vi "Close_Shot.vi"(4 "Far Shot":bool, 6 "Low_Goal":bool, 7 "Servo_Ref":T4={"ServoDeviceRef"={"DeviceStatus"={"status"=FALSE, "code"=0, "source"=""}, "PWM Channel"=enum."PWM 9", "DeadBand"={"Name"="Servo", "maxPositivePwm"=1770, "minPositivePwm"=1013, "centerPwm"=1007, "maxNegativePwm"=1000, "minNegativePwm"=243, "angularRange"=170}}, "error out"={"status"=FALSE, "code"=0, "source"=""}}, 8 "Close_Shot":bool) -> (0 "Shooter_Motor":dbl=1.0, 1 "Shooter_Arm":T5=enum."Out", 2 "Stage_Motor":T6=enum."Off", 3 "Shooter_Active":bool)   [LabVIEW 2015]
uses:
  Motor_Dir_Type_Def.ctl
  Arm_defense_Type_Def.ctl
  <vilib>/Rock Robotics/WPI/PWM/Servo/WPI_ServoDeviceRef.ctl
  <vilib>/Rock Robotics/SystemInterfaces/DIO/FPGA_DIOPWMChannel.ctl
  <vilib>/Rock Robotics/WPI/PWM/WPI_PWMDeadband.ctl
  Global_Var/Drive_Global.vi
  <vilib>/addons/control/pid/pid.llb/PID (DBL).vi
  <vilib>/Rock Robotics/Network Tables/NT Read Boolean.vi
  <vilib>/Rock Robotics/Network Tables/NT Read Number.vi
  <vilib>/Rock Robotics/Network Tables/NT Write Number.vi
  <vilib>/addons/control/pid/NI_PID_pid.lvlib
panel:
  in  "Low_Goal_WHeel_Speed":dbl=0.4
  in  "Far Angle":dbl=180.0
  in  "Dashboard_Enable":bool
  in  "Negate":bool=TRUE
  out "Waveform Chart":cluster{"Shooter_Speed":dbl, "output":dbl}(graph)={"Shooter_Speed"=0.85, "output"=0.6528102795997961}
  in  "PID gains":T7={"proportional gain (Kc)"=5.0, "integral time (Ti, min)"=0.01, "derivative time (Td, min)"=0.0} {"derivative time (Td, min)" format="%.3f"; "integral time (Ti, min)" format="%.3f"; "proportional gain (Kc)" format="%.3f"}
  in  "Shooter_Speed":dbl=0.85
  in  "Shooter_PID_Enable":bool=TRUE
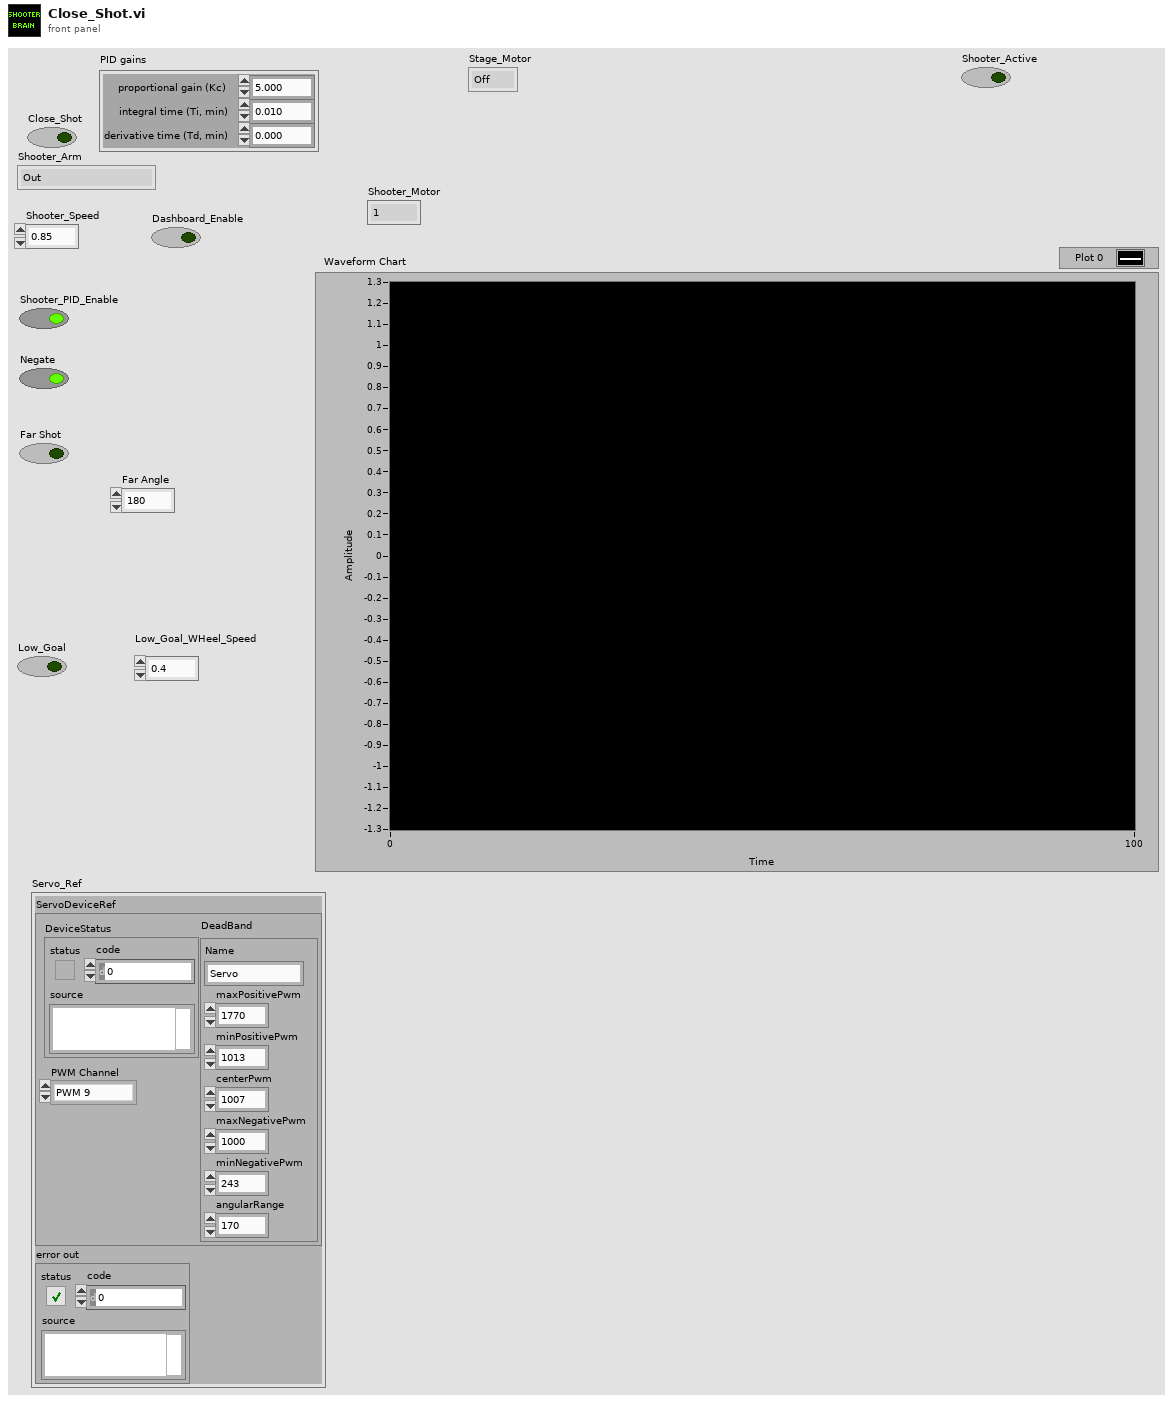
[diagram p1: front panel]
types:
  T1 = typedef "WPI_ServoDeviceRef.ctl" = cluster{"DeviceStatus":errorcluster, "PWM Channel":T2, "DeadBand":T3}
  T2 = typedef "FPGA_DIOPWMChannel.ctl" = enum8{"PWM 0", "PWM 1", "PWM 2", "PWM 3", "PWM 4", "PWM 5", "PWM 6", "PWM 7", "PWM 8", "PWM 9", "PWM MXP 0", "PWM MXP 1", "PWM MXP 2", "PWM MXP 3", "PWM MXP 4", "PWM MXP 5", "PWM MXP 6", "PWM MXP 7", "PWM MXP 8", "PWM MXP 9", "Invalid"}
  T3 = typedef "WPI_PWMDeadband.ctl" = cluster{"Name":string, "maxPositivePwm":i32, "minPositivePwm":i32, "centerPwm":i32, "maxNegativePwm":i32, "minNegativePwm":i32, "angularRange":u16}
  T4 = cluster{"ServoDeviceRef":T1, "error out":errorcluster}
  T5 = typedef "Arm_defense_Type_Def.ctl" = enum16{"Cheval de Frise", "Portcullis", "Out", "In", "Ball_Pickup"}
  T6 = typedef "Motor_Dir_Type_Def.ctl" = enum16{"In", "Out", "Off"}
  T7 = cluster{"proportional gain (Kc)":dbl, "integral time (Ti, min)":dbl, "derivative time (Td, min)":dbl}
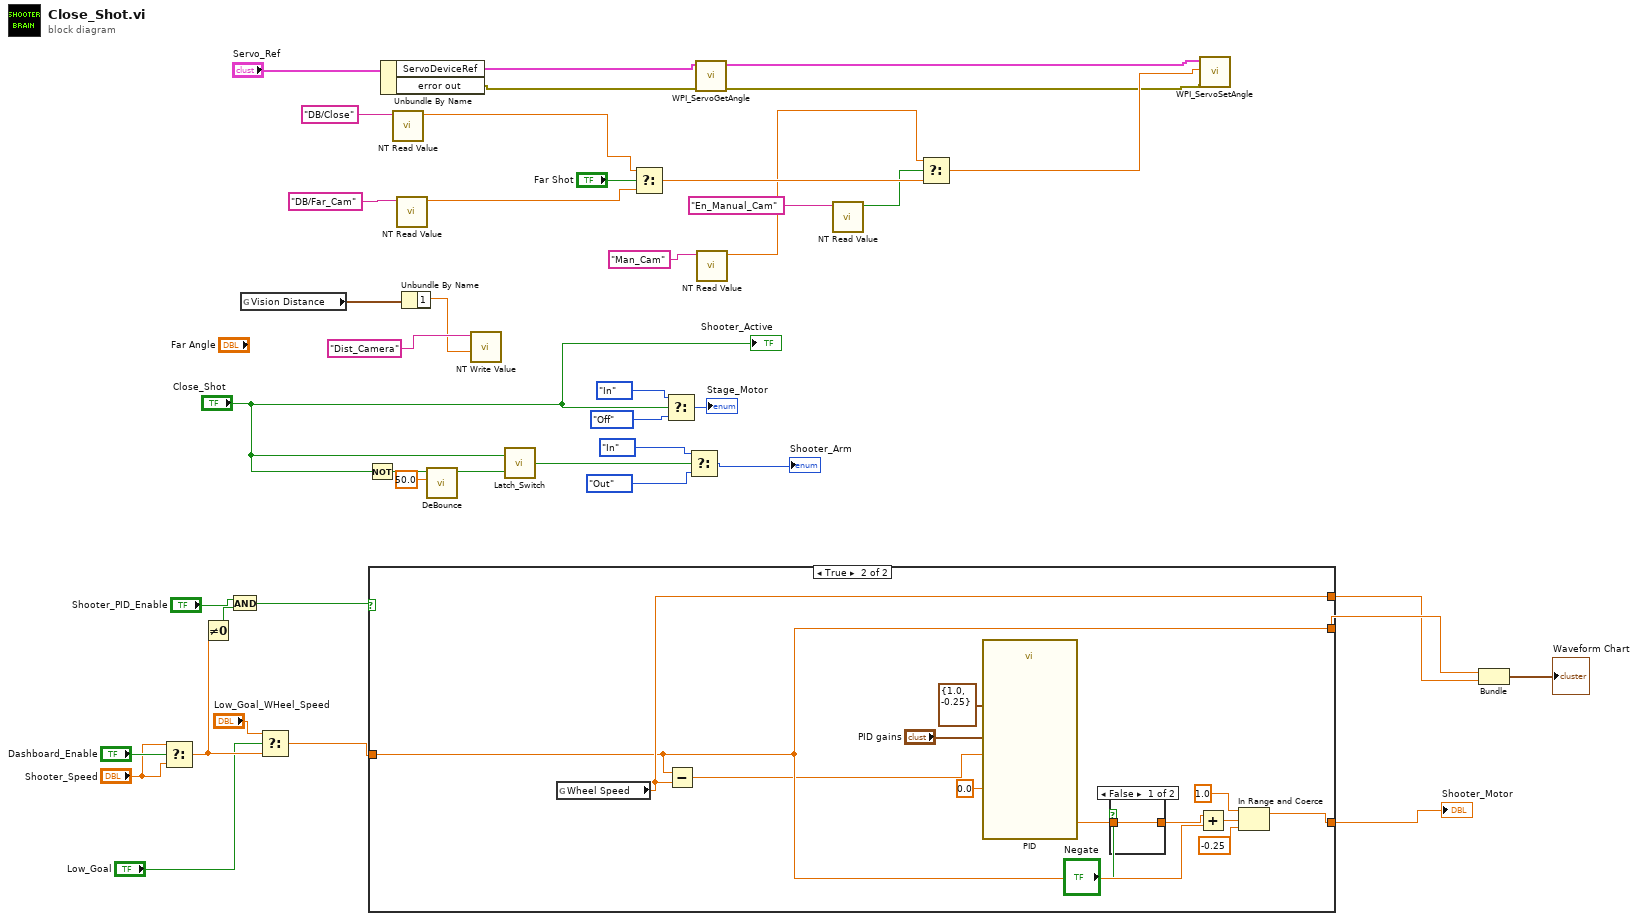
[diagram p0: block diagram]
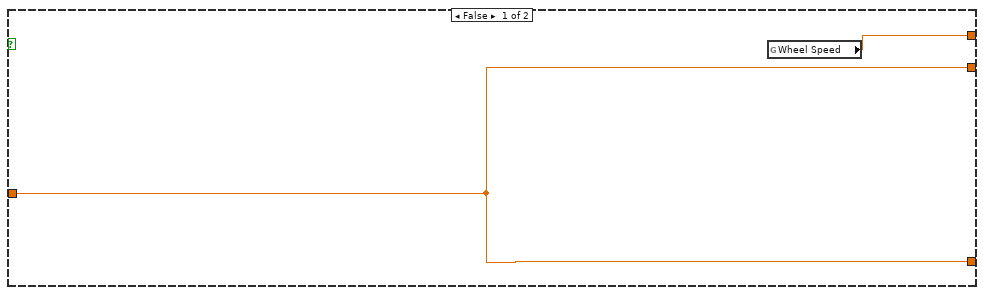
[diagram p2: hidden frame]
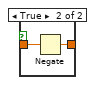
[diagram p3: hidden frame]
diagram:
  n1 = Select(t="Shooter_Speed", s="Dashboard_Enable", f="Shooter_Speed") -> (s? t:f=w20:dbl)
  n2 = Not Equal To 0?(x=w20) -> (x != 0?=w36:bool)
  n3 = And(x="Shooter_PID_Enable", y=w36) -> (x .and. y?=w35:bool)
  n4 = global read "Drive_Global.vi" "Vision Distance"() -> (w16:cluster{"1":dbl, "2":dbl, "3":dbl})
  n5 = Select(t="Low_Goal_WHeel_Speed", s="Low_Goal", f=w20) -> (s? t:f=w17:dbl)
  n6 = Not(x="Close_Shot") -> (.not. x?=w28:bool)
  n7 = case shown="True" w35 {
    tunnel: [w45 w53] -> w41
    tunnel: w17 -> [w45 w50]
    tunnel: [w45 w50] -> w42
    tunnel: [w44 w51] -> w34
    frame False {
      n8 = global read "Drive_Global.vi" "Wheel Speed"() -> (w44:dbl)
    }
    frame True {
      n9 = global read "Drive_Global.vi" "Wheel Speed"() -> (w51:dbl)
      n10 = Subtract(x=w50, y=w51) -> (x-y=w49:dbl)
      n11 = call-poly <vilib>:"PID.vi"("output range"=cluster{"output high":dbl, "output low":dbl} {"output high"=1.0, "output low"=-0.25}, "PID gains"="PID gains", "process variable"=w49, "setpoint"=0.0) -> ("output"=w48:dbl)  [unwired: 6 in, 1 out]
      n12 = case shown="False" "Negate" {
        tunnel: w48 -> [w59 w61]
        tunnel: [w59 w60] -> w47
        frame False {
        }
        frame True {
          n13 = Negate(x=w61) -> (-x=w60:dbl)
        }
      }
      n14 = Add(x=w47, y=w50) -> (x+y=w56:dbl)
      n15 = In Range and Coerce(upper limit=1.0, x=w56, lower limit=-0.25) -> (coerced(x)=w53:dbl)  [unwired: 1 out]
    }
  }
  "Shooter_Motor" <- w41
  n16 = Unbundle By Name("Servo_Ref") -> ("ServoDeviceRef"=w22:T1, "error out"=w21:errorcluster)
  n17 = call-poly <vilib>:"NT Read Value.vi"("Name"="DB/Close" ("refnum name")) -> ("Numeric"=w6:dbl)  [unwired: 9 in, 1 out]
  n18 = call-poly <vilib>:"NT Read Value.vi"("Name"="DB/Far_Cam" ("refnum name")) -> ("Numeric"=w1:dbl)  [unwired: 9 in, 1 out]
  n19 = Unbundle By Name(w16) -> ("1"=w8:dbl)
  n20 = call "DeBounce.vi"("DB_Count"=50.0, "Value"=w28) -> ("BD_Value"=w29:bool)  [unwired: 9 in]
  n21 = call-poly <vilib>:"NT Write Value.vi"("Numeric"=w8, "Name"="Dist_Camera" ("refnum name")) -> ()  [unwired: 9 in, 1 out]
  n22 = call "Latch_Switch.vi"("Reset"=w29, "In"="Close_Shot") -> ("Out"=w26:bool)
  n23 = Select(t=w6, s="Far Shot", f=w1) -> (s? t:f=w14:dbl)
  n24 = Select(t=Motor_Dir_Type_Def."In" ("Motor"), s="Close_Shot", f=Motor_Dir_Type_Def."Off" ("Motor")) -> (s? t:f=→"Stage_Motor":T6)
  n25 = Select(t=Arm_defense_Type_Def."In" ("P1_Value"), s=w26, f=Arm_defense_Type_Def."Out" ("P1_Value")) -> (s? t:f=→"Shooter_Arm":T5)
  n26 = call <vilib>:"WPI_ServoGetAngle.vi"("ServoDeviceRef"=w22, "error in (no error)"=w21) -> ("ServoDeviceRef"=w5:T1, "error out"=w3:errorcluster)  [unwired: 6 in, 1 out]
  n27 = call-poly <vilib>:"NT Read Value.vi"("Name"="Man_Cam" ("refnum name")) -> ("Numeric"=w10:dbl)  [unwired: 9 in, 1 out]
  n28 = call-poly <vilib>:"NT Read Value.vi"("Name"="En_Manual_Cam" ("refnum name")) -> ("Boolean"=w13:bool)  [unwired: 9 in, 1 out]
  n29 = Select(t=w10, s=w13, f=w14) -> (s? t:f=w4:dbl)
  n30 = call <vilib>:"WPI_ServoSetAngle.vi"("error in (no error)"=w3, "Angle"=w4, "ServoDeviceRef"=w5) -> ()  [unwired: 7 in, 2 out]
  n31 = Bundle("Shooter_Speed"=w42, "Wheel Speed"=w34) -> (→"Waveform Chart":cluster{"Shooter_Speed":dbl, "Wheel Speed":dbl})  [unwired: 1 in]
  "Shooter_Active" <- "Close_Shot"
